vi "dfd_Maxflat Create Param.vi"(9 "denominator order":i32=2, 10 "normalized fc":dbl=0.2, 11 "symmetric FIR ? (T)":bool) -> (2 "H0":dbl, 3 "x0":dbl=0.49999999999999994)   [LabVIEW 2017, in "NI_DigFilter_Design.lvlib"]
doc: "Creates the parameter for build polynomial."
uses:
  <vilib>/addons/Digital Filter Design/NI_DigFilter_Design.lvlib
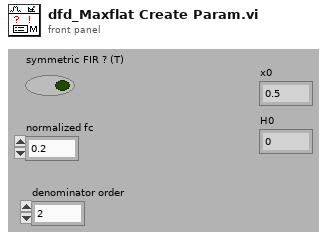
[diagram p1: front panel]
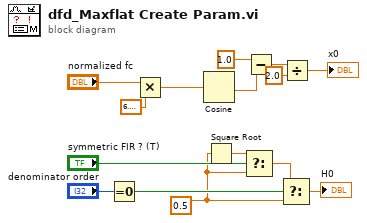
[diagram p0: block diagram]
diagram:
  w3 = 0.5
  n1 = Equal To 0?(x="denominator order") -> (x = 0?=w6:bool)
  n2 = Multiply(x="normalized fc", y=6.283185307179586) -> (x*y=w9:dbl)
  n3 = Cosine(x=w9) -> (cos(x)=w13:dbl)
  n4 = Square Root(x=w3) -> (sqrt(x)=w4:dbl)
  n5 = Select(t=w4, s="symmetric FIR ? (T)", f=w3) -> (s? t:f=w2:dbl)
  n6 = Subtract(x=1.0, y=w13) -> (x-y=w14:dbl)
  n7 = Select(t=w2, s=w6, f=w3) -> (s? t:f=→"H0":dbl)
  n8 = Divide(x=w14, y=2.0) -> (x/y=→"x0":dbl)
